vi "Draw Glyph.vi"(5 "Transform (Center)":refnum<class "Transform.lvclass">, 6 "Colors":T1={"Front"={"Color"=0, "Alpha"=255}, "Back"={"Color"=16448250, "Alpha"=255}}, 7 "Font (System)":refnum<class "Font Settings.lvclass">, 8 "error in (no error)":errorcluster, 9 "codepoint":u32, 10 "Glyph Drawer in":refnum<class "Glyph Drawer.lvclass">, 11 "Glyph Canvas in":refnum<class "Glyph Canvas.lvclass">) -> (0 "error out":errorcluster, 3 "Glyph Canvas out":refnum<class "Glyph Canvas.lvclass">)   [LabVIEW 2023, in "Font Glyph Drawer Interface.lvlib" / "Glyph Canvas.lvclass"]
uses:
  Glyph Canvas.lvclass
  Glyph Drawer/Glyph Drawer.lvclass
  Transform/Transform.lvclass
  Font Settings/Font Settings.lvclass
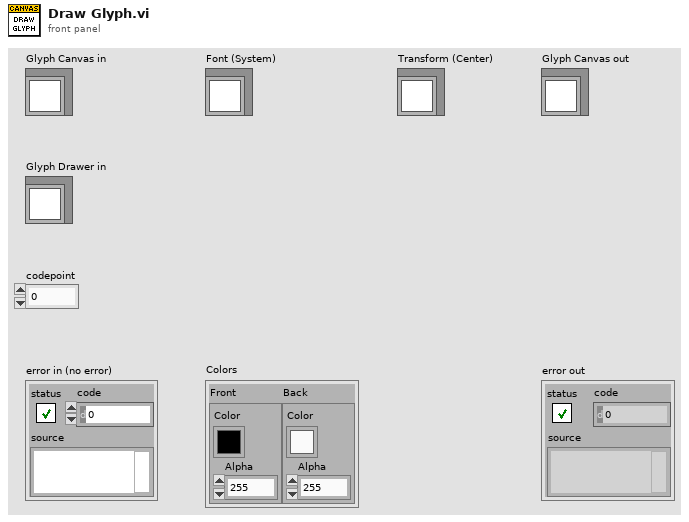
[diagram p1: front panel]
types:
  T1 = cluster{"Front":cluster{"Color":u32, "Alpha":u8}, "Back":cluster{"Color":u32, "Alpha":u8}}
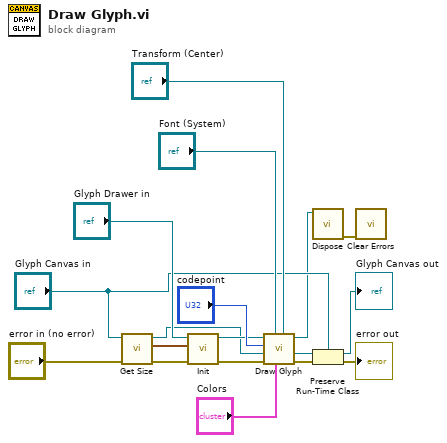
[diagram p0: block diagram]
diagram:
  n1 = call-dynamic "Get Size.vi"("error in (no error)"="error in (no error)", "Glyph Destination in"="Glyph Canvas in") -> ("error out"=w6:errorcluster, "Size"=w4:cluster{"Width":u16, "Height":u16}, "Glyph Destination out"=w5:refnum<class "Glyph Canvas.lvclass">)  [unwired: 7 in]
  n2 = call-dynamic "Init.vi"("error in (no error)"=w6, "Size"=w4, "Glyph Drawer in"="Glyph Drawer in") -> ("error out"=w9:errorcluster, "Glyph Drawer out"=w7:refnum<class "Glyph Drawer.lvclass">)  [unwired: 7 in]
  n3 = call-dynamic "Draw Glyph.vi"("Transform (Center)"="Transform (Center)", "Colors"="Colors", "Font (System)"="Font (System)", "error in (no error)"=w9, "Destination"=w5, "codepoint"="codepoint", "Glyph Drawer in"=w7) -> ("error out"=w17:errorcluster, "Destination Out"=w11:refnum<class "Glyph Canvas.lvclass">, "Glyph Drawer out"=w2:refnum<class "Glyph Drawer.lvclass">)  [unwired: 2 in]
  n4 = call-dynamic "Dispose.vi"("Glyph Drawer in"=w2) -> ("error out"=w1:errorcluster)  [unwired: 10 in]
  n5 = Preserve Run-Time Class(object in=w11, error in=w17, 2:"Glyph Canvas in") -> (object out=→"Glyph Canvas out":refnum<class "Glyph Canvas.lvclass">, error out=→"error out":errorcluster)
  n6 = call <vilib>:"Clear Errors.vi"("error in (no error)"=w1) -> ()  [unwired: 5 in, 2 out]
